vi "Vending Machine.vi"() -> ()   [LabVIEW 2020]
doc: "This VI simulates the functionality of the vending mechine"
uses:
  Controller/Product Select.ctl
  Controller/Main Controller.ctl
  Controller/Queue Controller.ctl
  Controller/Main data cluster.ctl
  Controller/File Operation Controller.ctl
panel:
  in  "error in":errorcluster
  out "error out":errorcluster
  out "Dispensing":bool
  out "Elapsed Time":dbl format="%.1g"
  in  "Selection Buttons":T1
  in  "Deposit":bool
  out "Change Returned":string="$0.00"
  in  "Coin Return":bool
  out "Amount Deposited":string="$0.00"
  in  "Exit":bool
  out "Products":T2[][](array[typedef])
  # "Vending Panel"
  # "Control Panel"
  # "4"
  # "1"
  # "3"
  # "2"
  # "A"
  # "B"
  # "C"
  # "D"
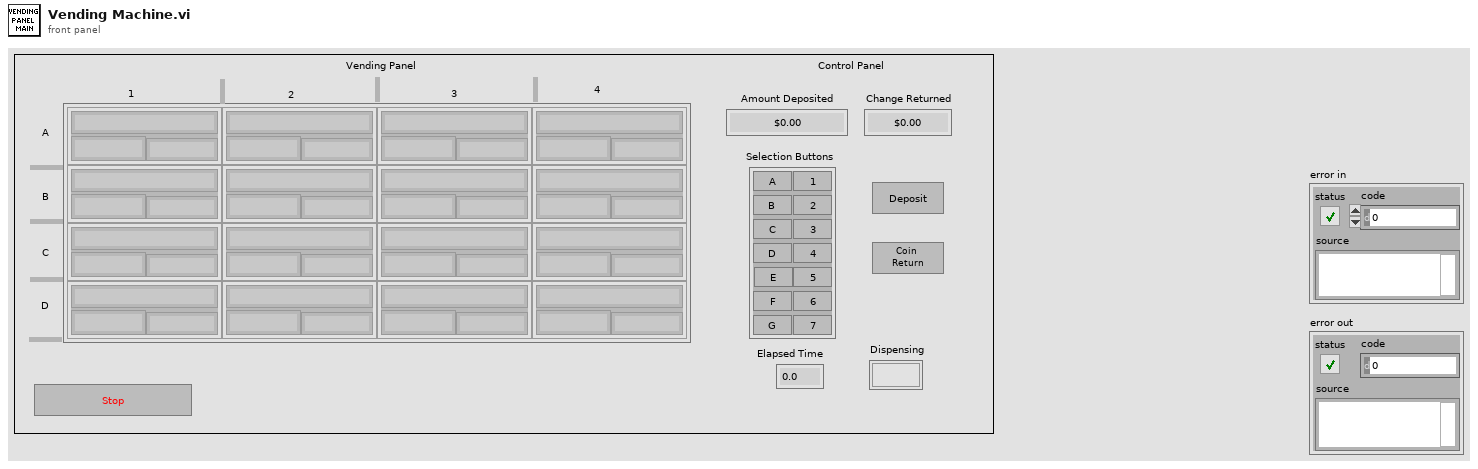
[diagram p1: front panel]
types:
  T1 = cluster{"AButton":bool, "BButton":bool, "CButton":bool, "DButton":bool, "EButton":bool, "FButton":bool, "GButton":bool, "1Button":bool, "2Button":bool, "3Button":bool, "4Button":bool, "5Button":bool, "6Button":bool, "7Button":bool}
  T2 = typedef "Product Select.ctl" = cluster{"Product Name":string, "Product Cost":string, "Inventory":string}
  T3 = typedef "Main data cluster.ctl" = cluster{"Amount Deposited":string, "Change Returned":string, "Dispensing":bool, "Elapsed Time":dbl, "Deposit":bool, "Coin Return":bool, "Exit":bool, "Selection Buttons":cluster{"AButton":bool, "BButton":bool, "CButton":bool, "DButton":bool, "EButton":bool, "FButton":bool, "GButton":bool, "1Button":bool, "2Button":bool, "3Button":bool, "4Button":bool, "5Button":bool, "6Button":bool, "7Button":bool}, "Products":T2[][], "program cluster":cluster{"is char btn":bool, "is num btn":bool, "is timer":bool, "depo amt":string, "i index":i32, "j index":i32, "timer val":u32}, "memory":cluster{"name":string, "price":string, "quantity":string}, "change return memory":string}
  T4 = typedef "Queue Controller.ctl" = enum16{"obtain queue", "enqueue", "dequeue", "enstack", "release que", "get queue stat"}
  T5 = typedef "Main Controller.ctl" = enum16{"init", "poll", "read file", "update md cluster ", "precheck", "display", "Calculate", "timer", "update file", "reset", "error", "exit"}
  T6 = cluster{"name":string, "price":string, "quantity":string}
  T7 = cluster{"is char btn":bool, "is num btn":bool, "is timer":bool, "depo amt":string, "i index":i32, "j index":i32, "timer val":u32}
  T8 = typedef "File Operation Controller.ctl" = enum16{"read", "write"}
  T9 = typedef "Product controller.ctl" = cluster{"name":string, "price":string, "quantity ":string}
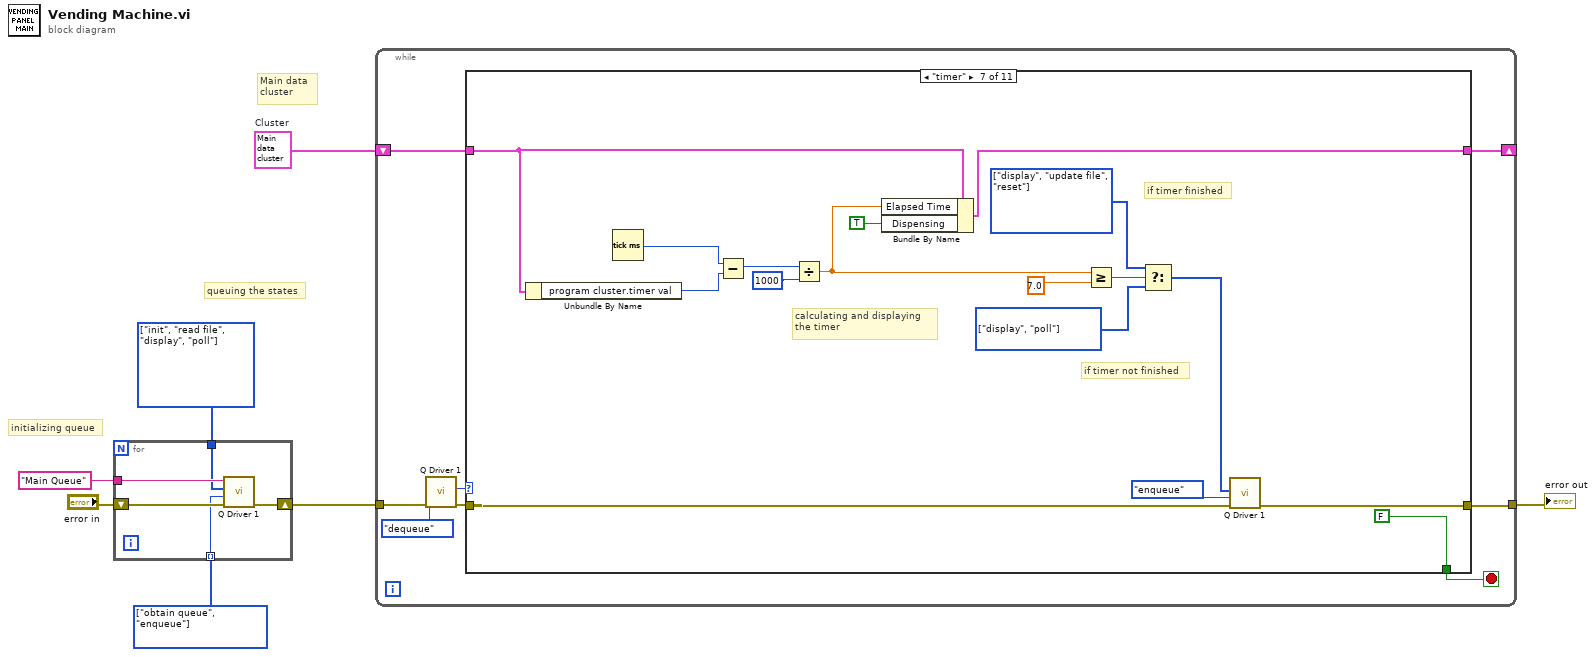
[diagram p0: block diagram]
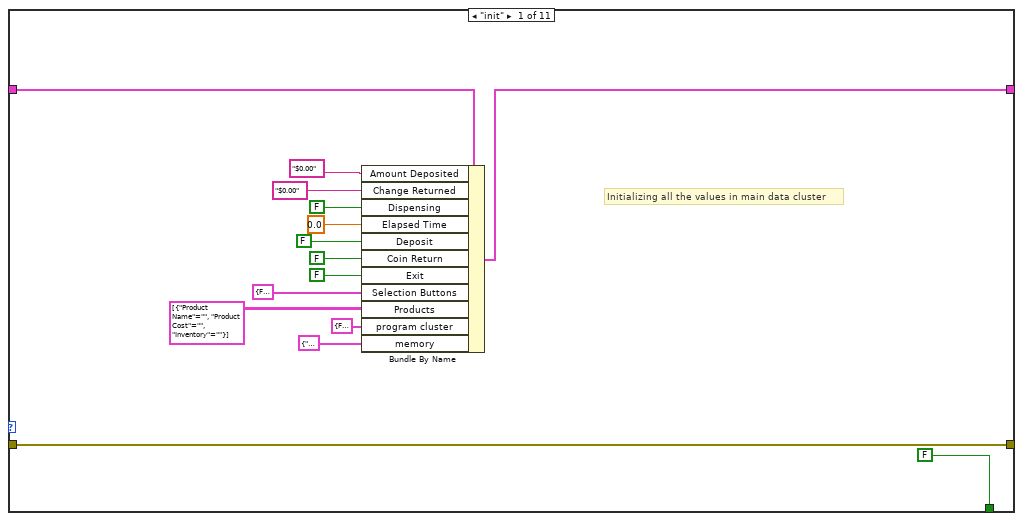
[diagram p2: hidden frame]
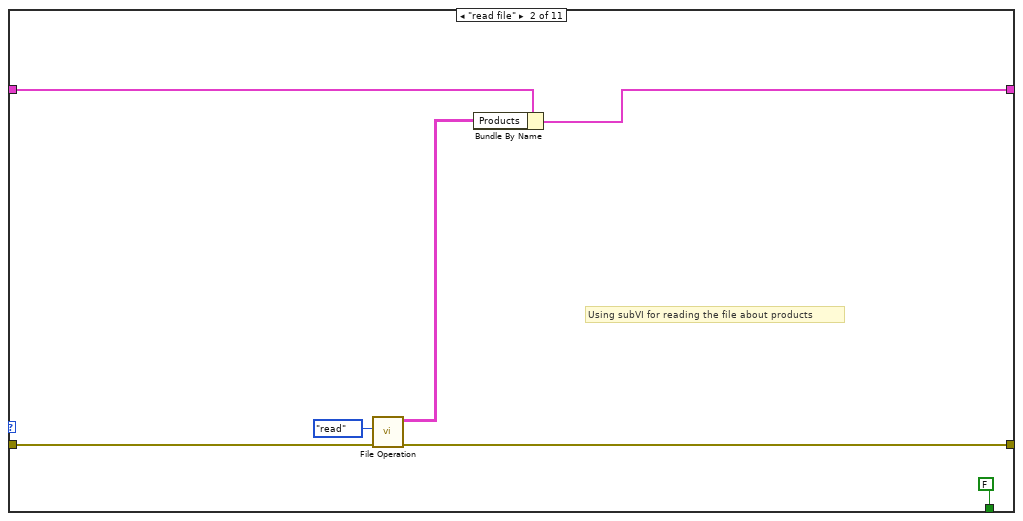
[diagram p3: hidden frame]
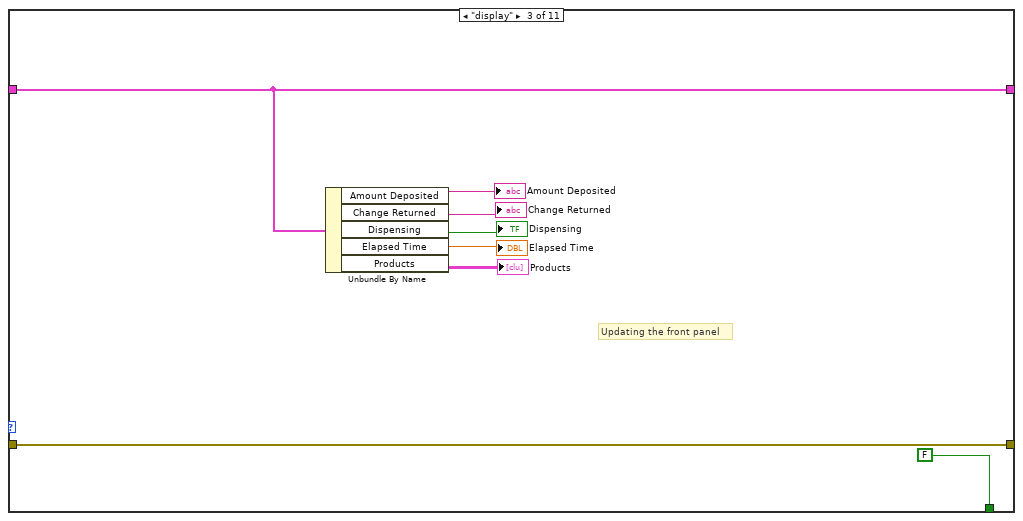
[diagram p4: hidden frame]
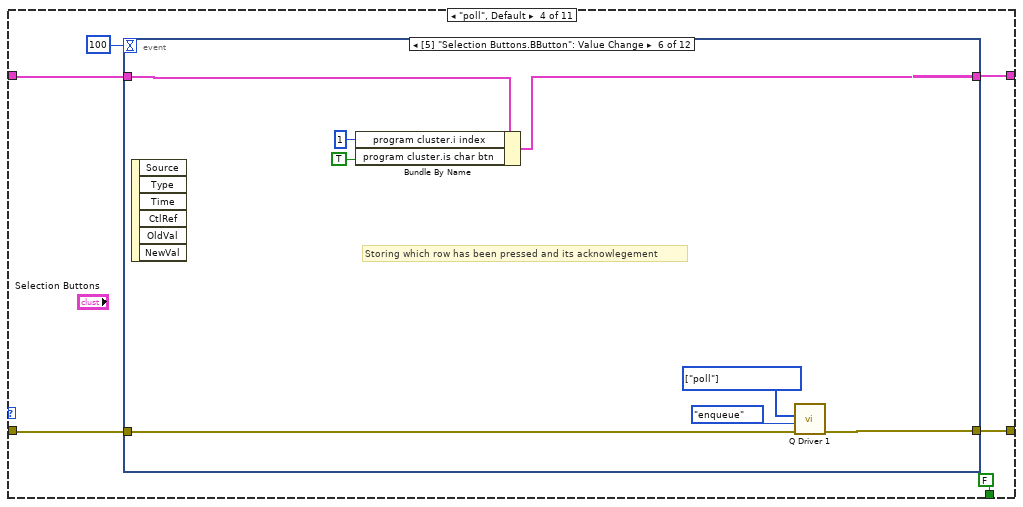
[diagram p5: hidden frame]
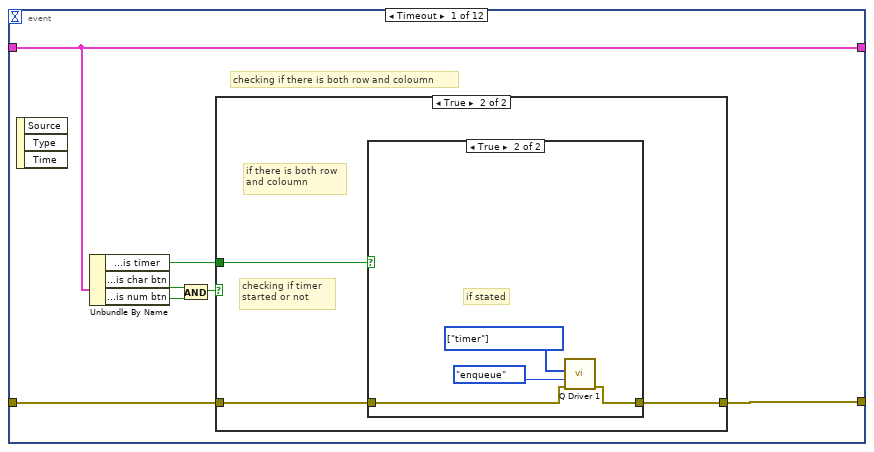
[diagram p6: hidden frame]
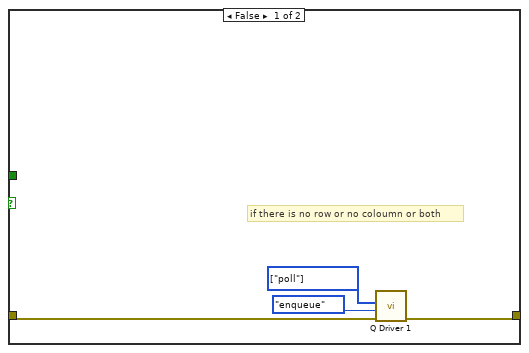
[diagram p7: hidden frame]
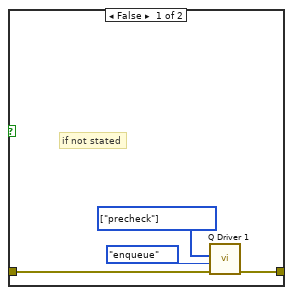
[diagram p8: hidden frame]
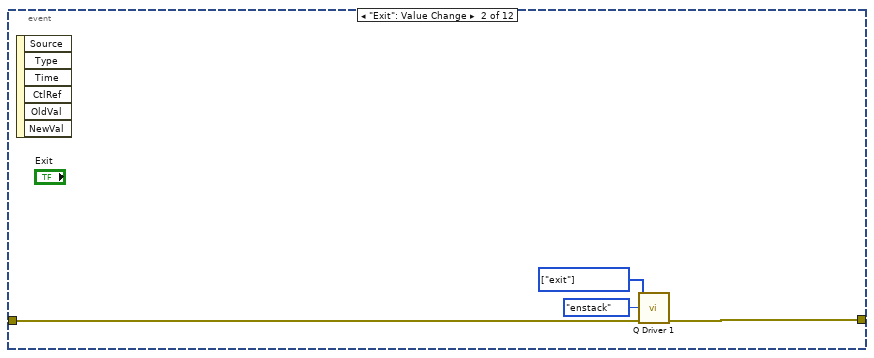
[diagram p9: hidden frame]
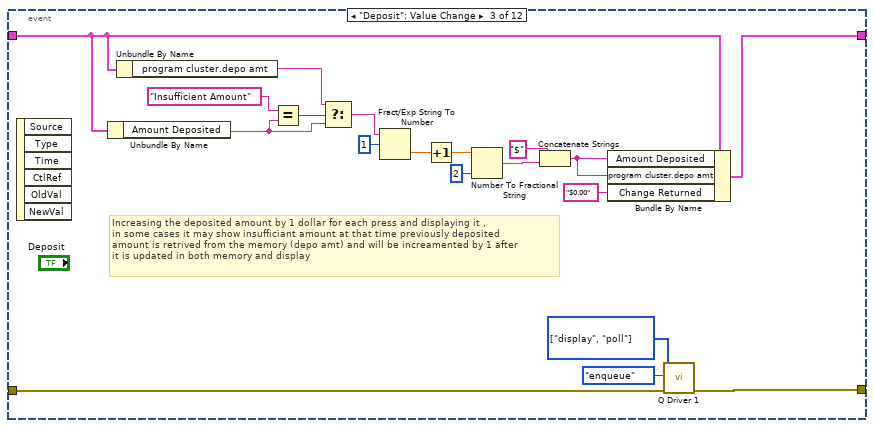
[diagram p10: hidden frame]
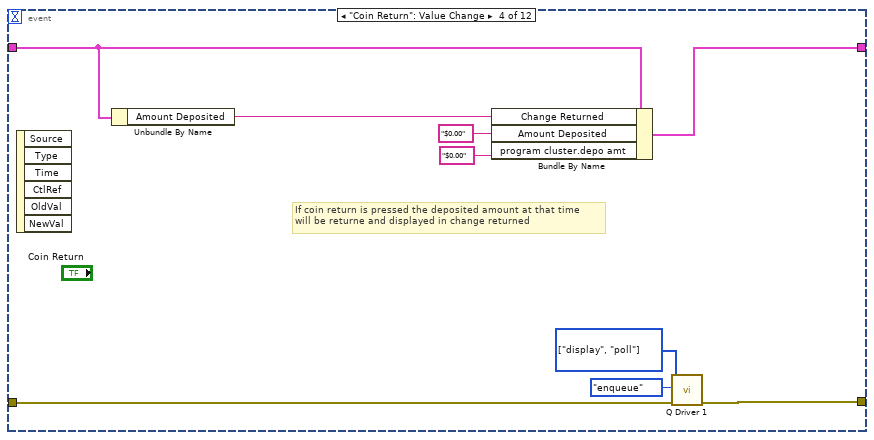
[diagram p11: hidden frame]
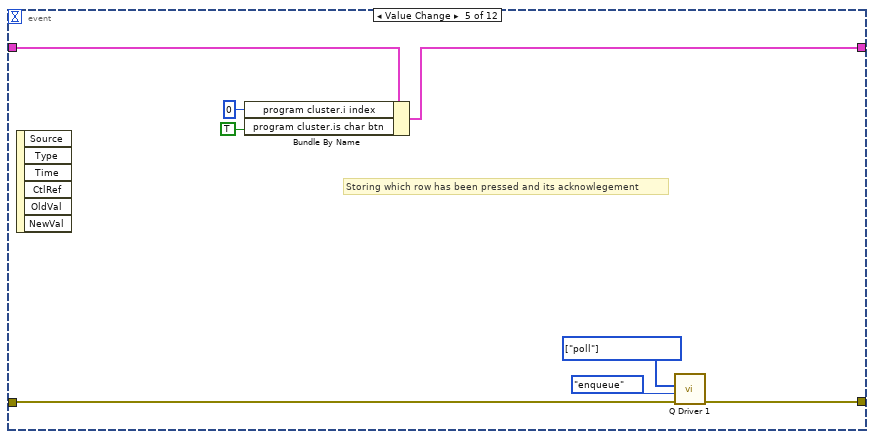
[diagram p12: hidden frame]
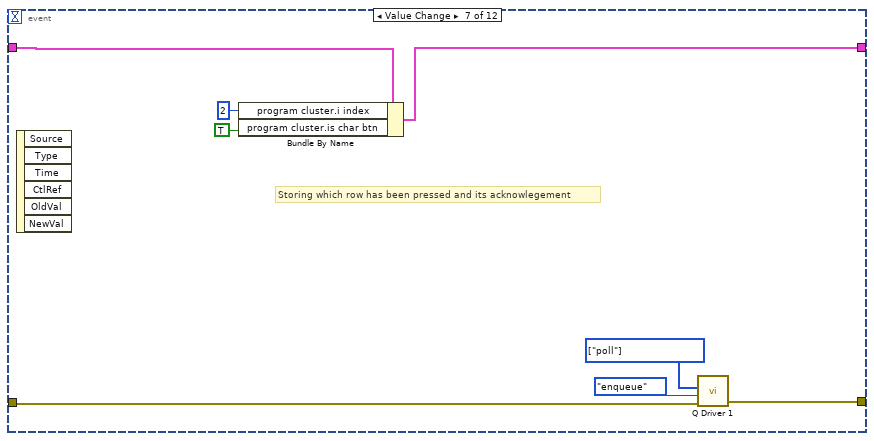
[diagram p13: hidden frame]
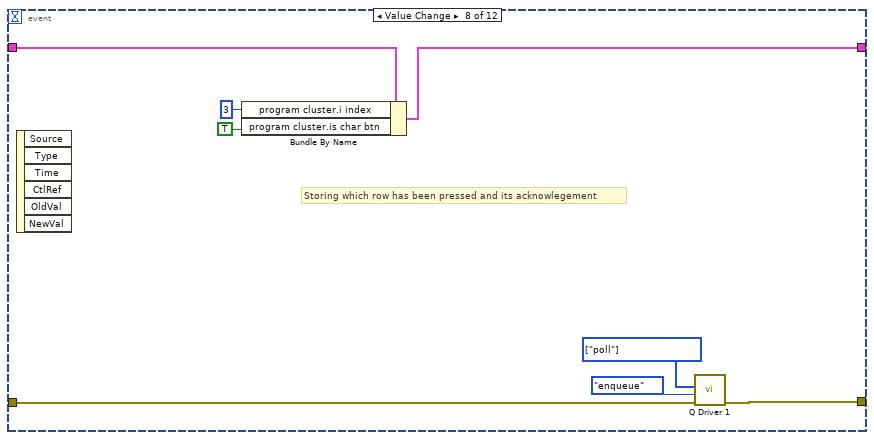
[diagram p14: hidden frame]
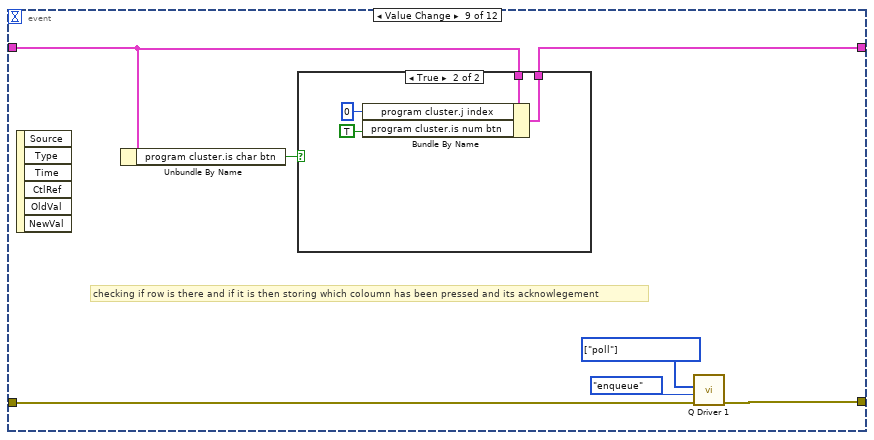
[diagram p15: hidden frame]
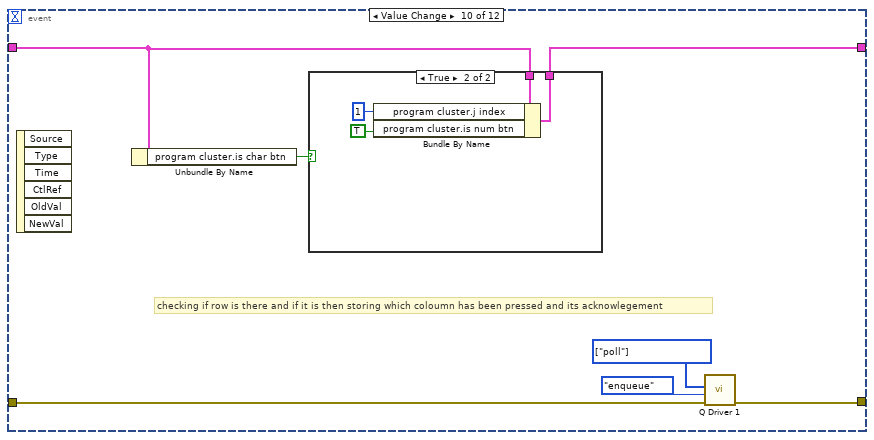
[diagram p17: hidden frame]
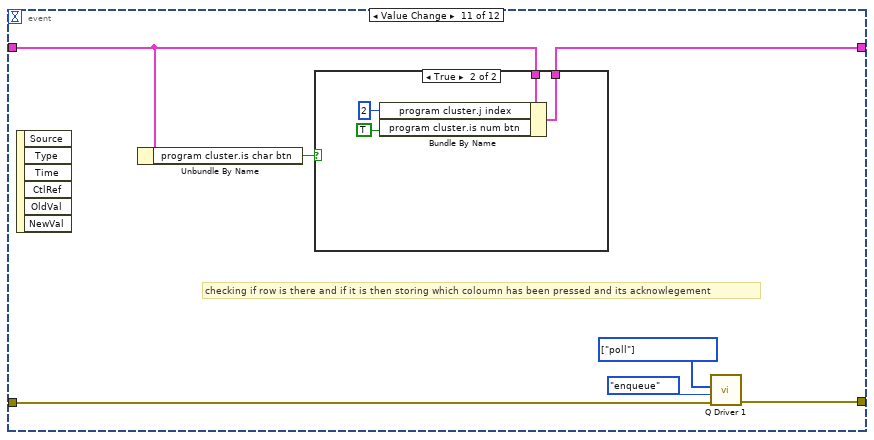
[diagram p19: hidden frame]
diagram:
  w1 = T3 {"Amount Deposited"="$0.00", "Change Returned"="$0.00", "Dispensing"=FALSE, "Elapsed Time"=0.0, "Deposit"=FALSE, "Coin Return"=FALSE, "Exit"=FALSE, "Selection Buttons"={"AButton"=FALSE, "BButton"=FALSE, "CButton"=FALSE, "DButton"=FALSE, "EButton"=FALSE, "FButton"=FALSE, "GButton"=FALSE, "1Button"=FALSE, "2Button"=FALSE, "3Button"=FALSE, "4Button"=FALSE, "5Button"=FALSE, "6Button"=FALSE, "7Button"=FALSE}, "Products"=[], "program cluster"={"is char btn"=FALSE, "is num btn"=FALSE, "is timer"=FALSE, "depo amt"="", "i index"=0, "j index"=0, "timer val"=0}, "memory"={"name"="", "price"="", "quantity"=""}, "change return memory"=""}  # Cluster
  w2 = T4[] [enum."obtain queue", enum."enqueue"] items=["obtain queue", "enqueue", "dequeue", "enstack", "release que", "get queue stat"]
  w3 = T5[] [enum."init", enum."read file", enum."display", enum."poll"] items=["init", "poll", "read file", "update md cluster ", "precheck", "display", "Calculate", "timer", "update file", "reset", "error", "exit"] ("EnQ/Enstack")
  # "Main data \ncluster"
  # "queuing the states"
  # "initializing queue"
  n1 = for {
    shift-right: [w11] -> w6
    shift-left: "error in" -> [w12]
    tunnel: "Main Queue" ("name") -> [w10]
    tunnel: w3 -> [w9]
    tunnel: w2 -> [w8] mode=indexing
    n2 = call "Q Driver 1.vi"("error in"=w12, "Enum"=w8, "EnQ/Enstack"=w9, "name"=w10) -> ("error out"=w11:errorcluster)  [unwired: 5 in, 2 out]
  }
  n3 = while {
    tunnel: w6 -> [w19]
    tunnel: [w20] -> w5
    shift-right: [w14] -> _
    shift-left: w1 -> [w15]
    stop <- w13 stop-if-true
    n4 = call "Q Driver 1.vi"("error in"=w19, "Enum"=Queue_Controller."dequeue") -> ("error out"=w18:errorcluster, "DQ ele"=w16:T5)  [unwired: 7 in, 1 out]
    n5 = case shown="\"timer\"" w16 {
      tunnel: w18 -> [w35 w41 w50 w55 w199 w261 w270 w287 w292 w310 w313]
      tunnel: [w35 w40 w50 w52 w198 w261 w269 w286 w291 w306 w313] -> w20
      tunnel: w15 -> [w34 w39 w49 w54 w193 w255 w265 w288 w300 w309 w312]
      tunnel: [w33 w37 w49 w53 w200 w254 w263 w288 w295 w309 w312] -> w14
      tunnel: [FALSE FALSE FALSE FALSE FALSE FALSE FALSE FALSE FALSE FALSE TRUE] -> w13
      frame "init" {
        # "Initializing all the values in main data cluster"
        n6 = Bundle By Name(cluster=w34, "Amount Deposited"="$0.00", "Change Returned"="$0.00", "Dispensing"=FALSE, "Elapsed Time"=0.0, "Deposit"=FALSE, "Coin Return"=FALSE, "Exit"=FALSE, "Selection Buttons"=T1 {"AButton"=FALSE, "BButton"=FALSE, "CButton"=FALSE, "DButton"=FALSE, "EButton"=FALSE, "FButton"=FALSE, "GButton"=FALSE, "1Button"=FALSE, "2Button"=FALSE, "3Button"=FALSE, "4Button"=FALSE, "5Button"=FALSE, "6Button"=FALSE, "7Button"=FALSE}, "Products"=T2[][] [[{"Product Name"="", "Product Cost"="", "Inventory"=""}]], "program cluster"=T7 {"is char btn"=FALSE, "is num btn"=FALSE, "is timer"=FALSE, "depo amt"="", "i index"=0, "j index"=0, "timer val"=0}, "memory"=T6 {"name"="", "price"="", "quantity"=""}) -> (w33:T3)
      }
      frame "read file" {
        # "Using subVI for reading the file about products"
        n7 = call "File Operation.vi"("error in (no error)"=w41, "Enum"=File_Operation_Controller."read") -> ("error out"=w40:errorcluster, "Array"=w38:T9[][])  [unwired: 8 in]
        n8 = Bundle By Name(cluster=w39, "Products"=w38) -> (w37:T3)
      }
      frame "display" {
        # "Updating the front panel"
        n9 = Unbundle By Name(w49) -> ("Amount Deposited"=→"Amount Deposited":string, "Change Returned"=→"Change Returned":string, "Dispensing"=→"Dispensing":bool, "Elapsed Time"=→"Elapsed Time":dbl, "Products"=→"Products":T2[][])
      }
      frame "poll", Default {
        n10 = event shown="[5] \"Selection Buttons.BButton\": Value Change" {
          selector: _ -> [_ _ _ _ _ _ _ _ _ _ _ _]
          dyn-events: _ -> [_ _ _ _ _ _ _ _ _ _ _ _]
          timeout: 100 -> [_ _ _ _ _ _ _ _ _ _ _ _]
          tunnel: w55 -> [w60 w80 w99 w103 w112 w121 w127 w137 w144 w156 w168 w180]
          tunnel: w54 -> [w58 _ w87 w109 w118 w122 w130 w138 w148 w158 w170 w182]
          tunnel: [w58 _ w86 w110 w116 w120 w129 w135 w149 w157 w169 w181] -> w53
          tunnel: [w59 w79 w98 w102 w111 w119 w128 w136 w143 w155 w167 w179] -> w52
          event Timeout {
            # "checking if there is both row and coloumn"
            n11 = event-data() -> ()  [unwired: 1 in, 3 out]
            n12 = Unbundle By Name(w58) -> ("program cluster.is timer"=w57:bool, "program cluster.is char btn"=w62:bool, "program cluster.is num btn"=w63:bool)
            n13 = And(x=w62, y=w63) -> (x .and. y?=w61:bool)
            n14 = case shown="True" w61 {
              tunnel: w60 -> [w65 w70]
              tunnel: [w64 w69] -> w59
              tunnel: w57 -> [_ w68]
              frame False {
                w67 = T5[] [enum."poll"] items=["init", "poll", "read file", "update md cluster ", "precheck", "display", "Calculate", "timer", "update file", "reset", "error", "exit"] ("EnQ/Enstack")
                # "if there is no row or no coloumn or both"
                n15 = call "Q Driver 1.vi"("error in"=w65, "Enum"=Queue_Controller."enqueue", "EnQ/Enstack"=w67) -> ("error out"=w64:errorcluster)  [unwired: 6 in, 2 out]
              }
              frame True {
                # "checking if timer \nstarted or not"
                # "if there is both row\nand coloumn"
                n16 = case shown="True" w68 {
                  tunnel: w70 -> [w72 w76]
                  tunnel: [w71 w75] -> w69
                  frame False {
                    w74 = T5[] [enum."precheck"] items=["init", "poll", "read file", "update md cluster ", "precheck", "display", "Calculate", "timer", "update file", "reset", "error", "exit"] ("EnQ/Enstack")
                    # "if not stated"
                    n17 = call "Q Driver 1.vi"("error in"=w72, "Enum"=Queue_Controller."enqueue", "EnQ/Enstack"=w74) -> ("error out"=w71:errorcluster)  [unwired: 6 in, 2 out]
                  }
                  frame True {
                    w78 = T5[] [enum."timer"] items=["init", "poll", "read file", "update md cluster ", "precheck", "display", "Calculate", "timer", "update file", "reset", "error", "exit"] ("EnQ/Enstack")
                    # "if stated"
                    n18 = call "Q Driver 1.vi"("error in"=w76, "Enum"=Queue_Controller."enqueue", "EnQ/Enstack"=w78) -> ("error out"=w75:errorcluster)  [unwired: 6 in, 2 out]
                  }
                }
              }
            }
          }
          event "Exit": Value Change {
            w82 = T5[] [enum."exit"] items=["init", "poll", "read file", "update md cluster ", "precheck", "display", "Calculate", "timer", "update file", "reset", "error", "exit"] ("EnQ/Enstack")
            n19 = event-data() -> ()  [unwired: 1 in, 6 out]
            n20 = call "Q Driver 1.vi"("error in"=w80, "Enum"=Queue_Controller."enstack", "EnQ/Enstack"=w82) -> ("error out"=w79:errorcluster)  [unwired: 6 in, 2 out]
          }
          event "Deposit": Value Change {
            w101 = T5[] [enum."display", enum."poll"] items=["init", "poll", "read file", "update md cluster ", "precheck", "display", "Calculate", "timer", "update file", "reset", "error", "exit"] ("EnQ/Enstack")
            # "Increasing the deposited amount by 1 dollar for each press and displaying it , \nin some cases it may show insufficiant amount at that time previously deposited \namount is retrived from the memory (depo amt) and will be increamented by 1 after \nit is updated in both memory and display"
            n21 = event-data() -> ()  [unwired: 1 in, 6 out]
            n22 = Unbundle By Name(w87) -> ("Amount Deposited"=w95:string)
            n23 = Unbundle By Name(w87) -> ("program cluster.depo amt"=w94:string)
            n24 = Equal?(x="Insufficient Amount", y=w95) -> (x = y?=w96:bool)
            n25 = Select(t=w94, s=w96, f=w95) -> (s? t:f=w93:string)
            n26 = Fract/Exp String To Number(string=w93, offset=1) -> (number=w92:dbl)  [unwired: 2 in, 1 out]
            n27 = Increment(x=w92) -> (x+1=w89:dbl)
            n28 = Number To Fractional String(number=w89, precision (6)=i16 2) -> (F-format string=w90:string)  [unwired: 2 in]
            n29 = Concatenate Strings("$" ("string"), w90) -> (w85:string)
            n30 = Bundle By Name(cluster=w87, "Amount Deposited"=w85, "program cluster.depo amt"=w85, "Change Returned"="$0.00") -> (w86:T3)
            n31 = call "Q Driver 1.vi"("error in"=w99, "Enum"=Queue_Controller."enqueue", "EnQ/Enstack"=w101) -> ("error out"=w98:errorcluster)  [unwired: 6 in, 2 out]
          }
          event "Coin Return": Value Change {
            w105 = T5[] [enum."display", enum."poll"] items=["init", "poll", "read file", "update md cluster ", "precheck", "display", "Calculate", "timer", "update file", "reset", "error", "exit"] ("EnQ/Enstack")
            # "If coin return is pressed the deposited amount at that time \nwill be returne and displayed in change returned"
            n32 = event-data() -> ()  [unwired: 1 in, 6 out]
            n33 = Unbundle By Name(w109) -> ("Amount Deposited"=w108:string)
            n34 = Bundle By Name(cluster=w109, "Change Returned"=w108, "Amount Deposited"="$0.00", "program cluster.depo amt"="$0.00") -> (w110:T3)
            n35 = call "Q Driver 1.vi"("error in"=w103, "Enum"=Queue_Controller."enqueue", "EnQ/Enstack"=w105) -> ("error out"=w102:errorcluster)  [unwired: 6 in, 2 out]
          }
          event "Selection Buttons.AButton": Value Change {
            w114 = T5[] [enum."poll"] items=["init", "poll", "read file", "update md cluster ", "precheck", "display", "Calculate", "timer", "update file", "reset", "error", "exit"] ("EnQ/Enstack")
            # "Storing which row has been pressed and its acknowlegement"
            n36 = event-data() -> ()  [unwired: 1 in, 6 out]
            n37 = Bundle By Name(cluster=w118, "program cluster.i index"=0, "program cluster.is char btn"=TRUE) -> (w116:T3)
            n38 = call "Q Driver 1.vi"("error in"=w112, "Enum"=Queue_Controller."enqueue", "EnQ/Enstack"=w114) -> ("error out"=w111:errorcluster)  [unwired: 6 in, 2 out]
          }
          event "Selection Buttons.BButton": Value Change {
            w124 = T5[] [enum."poll"] items=["init", "poll", "read file", "update md cluster ", "precheck", "display", "Calculate", "timer", "update file", "reset", "error", "exit"] ("EnQ/Enstack")
            # "Storing which row has been pressed and its acknowlegement"
            n39 = event-data() -> ()  [unwired: 1 in, 6 out]
            n40 = Bundle By Name(cluster=w122, "program cluster.i index"=1, "program cluster.is char btn"=TRUE) -> (w120:T3)
            n41 = call "Q Driver 1.vi"("error in"=w121, "Enum"=Queue_Controller."enqueue", "EnQ/Enstack"=w124) -> ("error out"=w119:errorcluster)  [unwired: 6 in, 2 out]
          }
          event "Selection Buttons.CButton": Value Change {
            w132 = T5[] [enum."poll"] items=["init", "poll", "read file", "update md cluster ", "precheck", "display", "Calculate", "timer", "update file", "reset", "error", "exit"] ("EnQ/Enstack")
            # "Storing which row has been pressed and its acknowlegement"
            n42 = event-data() -> ()  [unwired: 1 in, 6 out]
            n43 = Bundle By Name(cluster=w130, "program cluster.i index"=2, "program cluster.is char btn"=TRUE) -> (w129:T3)
            n44 = call "Q Driver 1.vi"("error in"=w127, "Enum"=Queue_Controller."enqueue", "EnQ/Enstack"=w132) -> ("error out"=w128:errorcluster)  [unwired: 6 in, 2 out]
          }
          event "Selection Buttons.DButton": Value Change {
            w140 = T5[] [enum."poll"] items=["init", "poll", "read file", "update md cluster ", "precheck", "display", "Calculate", "timer", "update file", "reset", "error", "exit"] ("EnQ/Enstack")
            # "Storing which row has been pressed and its acknowlegement"
            n45 = event-data() -> ()  [unwired: 1 in, 6 out]
            n46 = Bundle By Name(cluster=w138, "program cluster.i index"=3, "program cluster.is char btn"=TRUE) -> (w135:T3)
            n47 = call "Q Driver 1.vi"("error in"=w137, "Enum"=Queue_Controller."enqueue", "EnQ/Enstack"=w140) -> ("error out"=w136:errorcluster)  [unwired: 6 in, 2 out]
          }
          event "Selection Buttons.1Button": Value Change {
            w146 = T5[] [enum."poll"] items=["init", "poll", "read file", "update md cluster ", "precheck", "display", "Calculate", "timer", "update file", "reset", "error", "exit"] ("EnQ/Enstack")
            # "checking if row is there and if it is then storing which coloumn has been pressed and its acknowlegement"
            n48 = event-data() -> ()  [unwired: 1 in, 6 out]
            n49 = Unbundle By Name(w148) -> ("program cluster.is char btn"=w147:bool)
            n50 = case shown="True" w147 {
              tunnel: w148 -> [w150 w153]
              tunnel: [w150 w152] -> w149
              frame False {
              }
              frame True {
                n51 = Bundle By Name(cluster=w153, "program cluster.j index"=0, "program cluster.is num btn"=TRUE ("program cluster.is char btn")) -> (w152:T3)
              }
            }
            n52 = call "Q Driver 1.vi"("error in"=w144, "Enum"=Queue_Controller."enqueue", "EnQ/Enstack"=w146) -> ("error out"=w143:errorcluster)  [unwired: 6 in, 2 out]
          }
          event "Selection Buttons.2Button": Value Change {
            w160 = T5[] [enum."poll"] items=["init", "poll", "read file", "update md cluster ", "precheck", "display", "Calculate", "timer", "update file", "reset", "error", "exit"] ("EnQ/Enstack")
            # "checking if row is there and if it is then storing which coloumn has been pressed and its acknowlegement"
            n53 = event-data() -> ()  [unwired: 1 in, 6 out]
            n54 = Unbundle By Name(w158) -> ("program cluster.is char btn"=w161:bool)
            n55 = case shown="True" w161 {
              tunnel: w158 -> [w162 w165]
              tunnel: [w162 w164] -> w157
              frame False {
              }
              frame True {
                n56 = Bundle By Name(cluster=w165, "program cluster.j index"=1, "program cluster.is num btn"=TRUE ("program cluster.is char btn")) -> (w164:T3)
              }
            }
            n57 = call "Q Driver 1.vi"("error in"=w156, "Enum"=Queue_Controller."enqueue", "EnQ/Enstack"=w160) -> ("error out"=w155:errorcluster)  [unwired: 6 in, 2 out]
          }
          event "Selection Buttons.3Button": Value Change {
            w172 = T5[] [enum."poll"] items=["init", "poll", "read file", "update md cluster ", "precheck", "display", "Calculate", "timer", "update file", "reset", "error", "exit"] ("EnQ/Enstack")
            # "checking if row is there and if it is then storing which coloumn has been pressed and its acknowlegement"
            n58 = event-data() -> ()  [unwired: 1 in, 6 out]
            n59 = Unbundle By Name(w170) -> ("program cluster.is char btn"=w173:bool)
            n60 = case shown="True" w173 {
              tunnel: w170 -> [w174 w177]
              tunnel: [w174 w176] -> w169
              frame False {
              }
              frame True {
                n61 = Bundle By Name(cluster=w177, "program cluster.j index"=2, "program cluster.is num btn"=TRUE ("program cluster.is char btn")) -> (w176:T3)
              }
            }
            n62 = call "Q Driver 1.vi"("error in"=w168, "Enum"=Queue_Controller."enqueue", "EnQ/Enstack"=w172) -> ("error out"=w167:errorcluster)  [unwired: 6 in, 2 out]
          }
          event "Selection Buttons.4Button": Value Change {
            w184 = T5[] [enum."poll"] items=["init", "poll", "read file", "update md cluster ", "precheck", "display", "Calculate", "timer", "update file", "reset", "error", "exit"] ("EnQ/Enstack")
            # "checking if row is there and if it is then storing which coloumn has been pressed and its acknowlegement"
            n63 = event-data() -> ()  [unwired: 1 in, 6 out]
            n64 = Unbundle By Name(w182) -> ("program cluster.is char btn"=w185:bool)
            n65 = case shown="True" w185 {
              tunnel: w182 -> [w186 w189]
              tunnel: [w186 w188] -> w181
              frame False {
              }
              frame True {
                n66 = Bundle By Name(cluster=w189, "program cluster.j index"=3, "program cluster.is num btn"=TRUE ("program cluster.is char btn")) -> (w188:T3)
              }
            }
            n67 = call "Q Driver 1.vi"("error in"=w180, "Enum"=Queue_Controller."enqueue", "EnQ/Enstack"=w184) -> ("error out"=w179:errorcluster)  [unwired: 6 in, 2 out]
          }
        }
      }
      frame "precheck" {
        # "check for stock"
        # "check for sufficient \nbalance"
        # "finding the selected product"
        # "the selected product is stored in the \nmemory fo future use"
        n68 = Unbundle By Name(w193) -> ("Amount Deposited"=w202:string, "Products"=w209:T2[][], "program cluster.i index"=w208:i32, "program cluster.j index"=w207:i32)
        n69 = Index Array(array=w209, index (row)=w208, index (col)=w207) -> (element=w192:T2)
        n70 = Unbundle By Name(w192) -> ("Product Cost"=w206:string, "Inventory"=w205:string)
        n71 = Bundle By Name(cluster=w193, "memory"=w192) -> (w191:T3)
        n72 = Fract/Exp String To Number(string=w202, offset=1) -> (number=w201:dbl)  [unwired: 2 in, 1 out]
        n73 = Fract/Exp String To Number(string=w206, offset=1) -> (number=w203:dbl)  [unwired: 2 in, 1 out]
        n74 = Equal?(x=w205, y="Sold Out") -> (x = y?=w197:bool)
        n75 = Greater Or Equal?(x=w201, y=w203) -> (x >= y?=w196:bool)
        n76 = case shown="False" w197 {
          tunnel: w191 -> [w213 w235]
          tunnel: [w212 w234] -> w200
          tunnel: w199 -> [w215 w241]
          tunnel: [w211 w240] -> w198
          tunnel: w196 -> [w214 _]
          frame False {
            # "if stock"
            n77 = case shown="False" w214 {
              tunnel: w215 -> [w218 w229]
              tunnel: w213 -> [w220 w232]
              tunnel: [w219 w232] -> w212
              tunnel: [w217 w228] -> w211
              frame False {
                w226 = T5[] [enum."display", enum."poll"] items=["init", "poll", "read file", "update md cluster ", "precheck", "display", "Calculate", "timer", "update file", "reset", "error", "exit"] ("EnQ/Enstack")
                # "if insufficient balance"
                n78 = Bundle By Name(cluster=w220, "Amount Deposited"="Insufficient Amount", "program cluster.is char btn"=FALSE, "program cluster.is num btn"=FALSE, "program cluster.i index"=0, "program cluster.j index"=0, "memory"=T6 {"name"="", "price"="", "quantity"=""}) -> (w219:T3)
                n79 = call "Q Driver 1.vi"("error in"=w218, "Enum"=Queue_Controller."enqueue", "EnQ/Enstack"=w226) -> ("error out"=w217:errorcluster)  [unwired: 6 in, 2 out]
              }
              frame True {
                w230 = T5[] [enum."Calculate", enum."timer"] items=["init", "poll", "read file", "update md cluster ", "precheck", "display", "Calculate", "timer", "update file", "reset", "error", "exit"] ("EnQ/Enstack")
                # "if sufficient balance"
                n80 = call "Q Driver 1.vi"("error in"=w229, "Enum"=Queue_Controller."enqueue", "EnQ/Enstack"=w230) -> ("error out"=w228:errorcluster)  [unwired: 6 in, 2 out]
              }
            }
          }
          frame True {
            w243 = T5[] [enum."poll"] items=["init", "poll", "read file", "update md cluster ", "precheck", "display", "Calculate", "timer", "update file", "reset", "error", "exit"] ("EnQ/Enstack")
            # "if no stock"
            n81 = Bundle By Name(cluster=w235, "program cluster.is char btn"=FALSE, "program cluster.is num btn"=FALSE, "program cluster.i index"=0, "program cluster.j index"=0, "memory"=T6 {"name"="", "price"="", "quantity"=""}) -> (w234:T3)
            n82 = call "Q Driver 1.vi"("error in"=w241, "Enum"=Queue_Controller."enqueue", "EnQ/Enstack"=w243) -> ("error out"=w240:errorcluster)  [unwired: 6 in, 2 out]
          }
        }
      }
      frame "Calculate" {
        # "Calculating the change and initiating the timerr"
        n83 = Unbundle By Name(w255) -> ("Amount Deposited"=w258:string, "memory"=w244:T6)
        n84 = Unbundle By Name(w244) -> ("price"=w259:string)
        n85 = Fract/Exp String To Number(string=w258, offset=1) -> (number=w257:dbl)  [unwired: 2 in, 1 out]
        n86 = Fract/Exp String To Number(string=w259, offset=1) -> (number=w256:dbl)  [unwired: 2 in, 1 out]
        n87 = Subtract(x=w257, y=w256) -> (x-y=w245:dbl)
        n88 = Number To Fractional String(number=w245, precision (6)=i16 2) -> (F-format string=w246:string)  [unwired: 2 in]
        n89 = Concatenate Strings("$" ("string"), w246) -> (w250:string)
        n90 = Tick Count (ms)() -> (millisecond timer value=w248:u32)
        n91 = Bundle By Name(cluster=w255, "change return memory"=w250, "program cluster.is timer"=TRUE, "program cluster.timer val"=w248) -> (w254:T3)
      }
      frame "timer" {
        w267 = T5[] [enum."display", enum."poll"] items=["init", "poll", "read file", "update md cluster ", "precheck", "display", "Calculate", "timer", "update file", "reset", "error", "exit"] ("EnQ/Enstack")
        w268 = T5[] [enum."display", enum."update file", enum."reset"] items=["init", "poll", "read file", "update md cluster ", "precheck", "display", "Calculate", "timer", "update file", "reset", "error", "exit"] ("EnQ/Enstack")
        # "if timer not finished"
        # "if timer finished"
        # "calculating and displaying \nthe timer"
        n92 = Unbundle By Name(w265) -> ("program cluster.timer val"=w276:u32)
        n93 = Tick Count (ms)() -> (millisecond timer value=w277:u32)
        n94 = Subtract(x=w277, y=w276) -> (x-y=w274:u32)
        n95 = Divide(x=w274, y=u32 1000) -> (x/y=w264:dbl)
        n96 = Bundle By Name(cluster=w265, "Elapsed Time"=w264, "Dispensing"=TRUE) -> (w263:T3)
        n97 = Greater Or Equal?(x=w264, y=7.0) -> (x >= y?=w272:bool)
        n98 = Select(t=w268, s=w272, f=w267) -> (s? t:f=w266:T5[])
        n99 = call "Q Driver 1.vi"("error in"=w270, "Enum"=Queue_Controller."enqueue", "EnQ/Enstack"=w266) -> ("error out"=w269:errorcluster)  [unwired: 6 in, 2 out]
      }
      frame "update file" {
        # "updates the file using subVI by prividing the input cluster \nand enum defing the operation also we decrementing the count \nin the input cluster"
        n100 = Unbundle By Name(w288) -> ("memory"=w279:T6)
        n101 = Unbundle By Name(w279) -> ("quantity"=w284:string)
        n102 = Decimal String To Number(string=w284) -> (number=w283:i32)  [unwired: 2 in, 1 out]
        n103 = Decrement(x=w283) -> (x-1=w282:i32)
        n104 = Number To Decimal String(number=w282) -> (decimal integer string=w281:string)  [unwired: 1 in]
        n105 = Bundle By Name(cluster=w279, "quantity"=w281) -> (w280:T6)
        n106 = call "File Operation.vi"("error in (no error)"=w287, "Enum"=File_Operation_Controller."write", "Cluster"=w280) -> ("error out"=w286:errorcluster)  [unwired: 7 in, 1 out]
      }
      frame "reset" {
        w294 = T5[] [enum."read file", enum."display", enum."poll"] items=["init", "poll", "read file", "update md cluster ", "precheck", "display", "Calculate", "timer", "update file", "reset", "error", "exit"] ("EnQ/Enstack")
        # "Resets back to initial state"
        n107 = Unbundle By Name(w300) -> ("change return memory"=w301:string)
        n108 = Bundle By Name(cluster=w300, "Amount Deposited"="$0.00", "Change Returned"=w301, "Dispensing"=FALSE, "Elapsed Time"=0.0, "program cluster"=T7 {"is char btn"=FALSE, "is num btn"=FALSE, "is timer"=FALSE, "depo amt"="", "i index"=0, "j index"=0, "timer val"=0}, "memory"=T6 {"name"="", "price"="", "quantity"=""}, "change return memory"="") -> (w295:T3)
        n109 = call "Q Driver 1.vi"("error in"=w292, "Enum"=Queue_Controller."enqueue", "EnQ/Enstack"=w294) -> ("error out"=w291:errorcluster)  [unwired: 6 in, 2 out]
      }
      frame "error" {
        w305 = T5[] [enum."poll"] items=["init", "poll", "read file", "update md cluster ", "precheck", "display", "Calculate", "timer", "update file", "reset", "error", "exit"] ("EnQ/Enstack")
        # "handles error"
        n110 = call <vilib>:"Clear Errors.vi"("error in (no error)"=w310) -> ("error out"=w307:errorcluster)  [unwired: 5 in, 1 out]
        n111 = call "Q Driver 1.vi"("error in"=w307, "Enum"=Queue_Controller."enqueue", "EnQ/Enstack"=w305) -> ("error out"=w306:errorcluster)  [unwired: 6 in, 2 out]
      }
      frame "exit" {
      }
    }
  }
  "error out" <- w5
